vi "no_overriding_method_warning.vi"(0 "Controller (in)":refnum<class "_Controller.lvclass">, 5 "error in (no error)":errorcluster) -> (14 "Controller (out)":refnum<class "_Controller.lvclass">, 17 "msg":string="The action '%s' for the referenced controller model '%s' is not currently supported in this version of the Arcus USB Communications driver.  \n\nHowever, refer to the ASCII Language Specification section of the %s controller documenation and the Examples section for issuing raw ASCII commands.   Any and ALL ASCII commands can be issued to the controller via the Send / Receive Command VI.\n\nIf the feature you are looking for appears to be too complicated to integrate into your project, please email us at 'info@kodintegrations.com' briefly desribing the action you're attempting to perform and the hardware you're controlling.", 19 "error out":errorcluster)   [LabVIEW 2020, in "common.lvlib"]
doc: "This is a warning routine placed in many of the top level \"Controller\" class abstract methods. If the User sees the message presented in this VI, then that suggests the abstract method they're attempting to execute does NOT have an overriding method available for their specific controller model.\n\nProduced By:\n\n<B>Kod Integrations, LLC</B>\n4835 Marianne Drive\nMount Airy, MD 21771\nhttp://www.kodintegrations.com\nemail: info@kodintegrations.com\nphone: (240) 687-1288"
uses:
  common.lvlib
  _Controller.lvclass
  _Controller.lvclass/_Controller.ctl
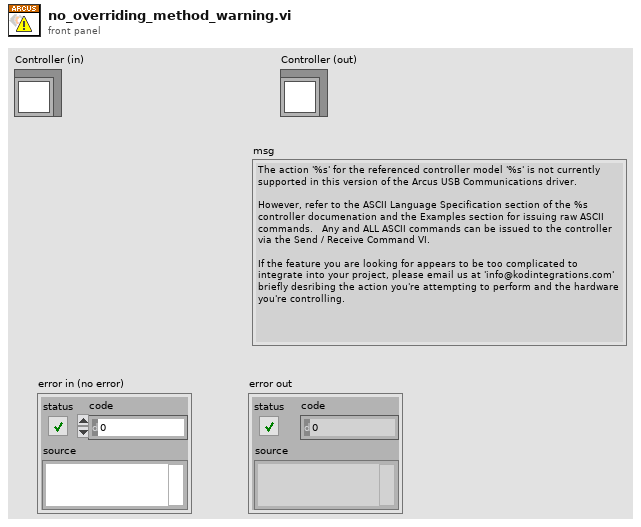
[diagram p1: front panel]
types:
  T1 = typedef "common.lvlib/models.ctl" = enum16{"<unrecognized>", "ACE-SDC", "ACE-SDE", "ACE-SXC", "ACE-SXE", "DMX-CAN", "DMX-J-SA", "DMX-K-SA", "DMX-UMD", "PMX-2ED-SA", "PMX-2EX-SA", "PMX-4CX-SA", "PMX-4EX-SA"}
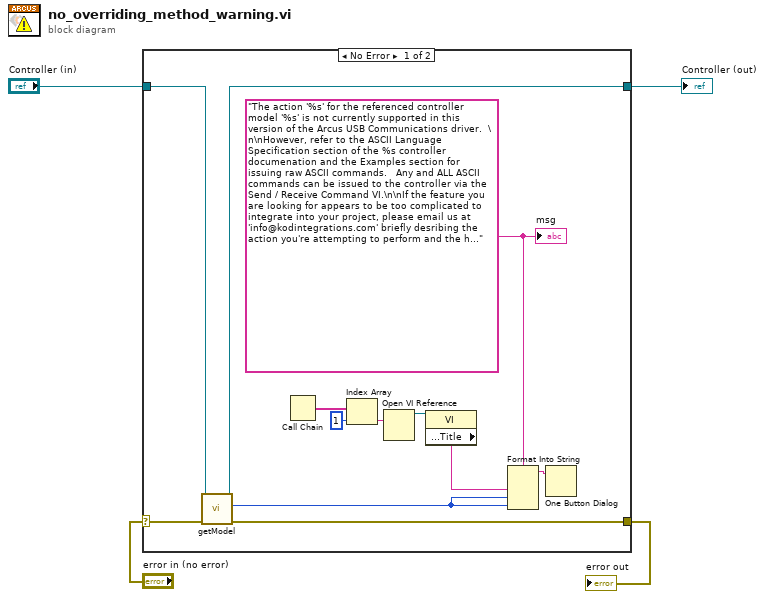
[diagram p0: block diagram]
diagram:
  n1 = case shown="No Error" "error in (no error)" {
    selector: "error in (no error)" -> [w6 w17]
    tunnel: "Controller (in)" -> [w15 w18]
    tunnel: [w14 w18] -> w3
    tunnel: [w5 w17] -> w1
    frame No Error {
      w8 = "The action '%s' for the referenced controller model '%s' is not currently supported in this version of the Arcus USB Communications driver.  \n\nHowever, refer to the ASCII Language Specification section of the %s controller documenation and the Examples section for issuing raw ASCII commands.   Any and ALL ASCII commands can be issued to the controller via the Send / Receive Command VI.\n\nIf the feature you are looking for appears to be too complicated to integrate into your project, please email us at 'info@kodintegrations.com' briefly desribing the action you're attempting to perform and the hardware you're controlling."
      n2 = call "getModel.vi"("error in (no error)"=w6, "reference (in)"=w15) -> ("error out"=w5:errorcluster, "model"=w7:T1, "reference (out)"=w14:refnum<class "_Controller.lvclass">)  [unwired: 7 in]
      n3 = Call Chain() -> (call chain=w13:string[])
      n4 = Index Array(array=w13, index=1) -> (element=w11:string)
      n5 = Open VI Reference(vi path=w11) -> (vi reference=w10:refnum<vi>)  [unwired: 5 in, 1 out]
      n6 = property class="VI"(reference=w10) -> ("Front Panel.Title"=w9:string)  [unwired: 1 in, 2 out]
      n7 = Format Into String(format string=w8, w9, w7, w7) -> (resulting string=w16:string)  [unwired: 2 in, 1 out]
      n8 = One Button Dialog(message=w16) -> ()  [unwired: 1 in, 1 out]
      "msg" <- w8
    }
    frame Error {
    }
  }
  "error out" <- w1
  "Controller (out)" <- w3
